vi "Open.vi"(7 "Path":path, 8 "error in (no error)":errorcluster, 10 "Operation":T1, 11 "Data in":refnum<class "Data.lvclass">) -> (0 "error out":errorcluster, 3 "Data out":refnum<class "Data.lvclass">)   [LabVIEW 2019, in "Data.lvclass"]
uses:
  Data.lvclass
  Typedefs/Operation--enum.ctl
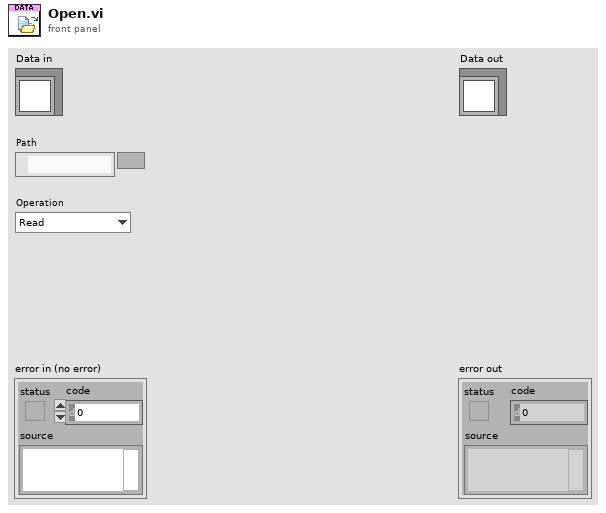
[diagram p1: front panel]
types:
  T1 = typedef "Data.lvclass/Operation--enum.ctl" = enum16{"Read", "Write", "Write + Append"}
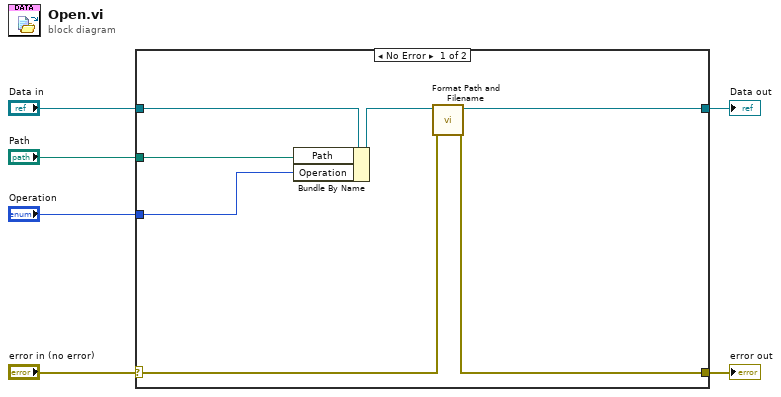
[diagram p0: block diagram]
diagram:
  n1 = case shown="No Error" "error in (no error)" {
    selector: "error in (no error)" -> [w8 w15]
    tunnel: [w7 w15] -> w5
    tunnel: [w9 w14] -> w3
    tunnel: "Data in" -> [w12 w14]
    tunnel: "Path" -> [w13 _]
    tunnel: "Operation" -> [w11 _]
    frame No Error {
      n2 = Bundle By Name(cluster=w12, "Path"=w13, "Operation"=w11) -> (w10:refnum<class "Data.lvclass">)
      n3 = call "Format Path and Filename.vi"("error in"=w8, "Data in"=w10) -> ("error out"=w7:errorcluster, "Data out"=w9:refnum<class "Data.lvclass">)  [unwired: 8 in]
    }
    frame Error {
    }
  }
  "error out" <- w5
  "Data out" <- w3
